vi "Init.vi"(8 "error in":errorcluster, 10 "File Path":path, 11 "XLS in":refnum<class "XLS.lvclass">) -> (0 "error out":errorcluster, 3 "XLS out":refnum<class "XLS.lvclass">)   [LabVIEW 2017, in "Report_lib.lvlib" / "XLS.lvclass"]
doc: "This method serves for Creating XLS file\nand Generate its filename"
uses:
  XLS.lvclass
  I:/TEMP/Source/Classes/Log/Log.lvclass
  Log/Log.lvclass/Log.ctl
  XLS.lvclass/XLS.ctl
  Log/Log.lvclass
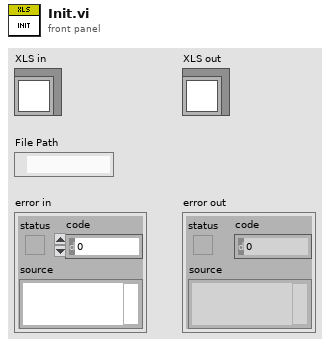
[diagram p1: front panel]
types:
  T1 = typedef "Log Data.ctl" = cluster{"File Path":path, "File Name":string, "File Ext":string}
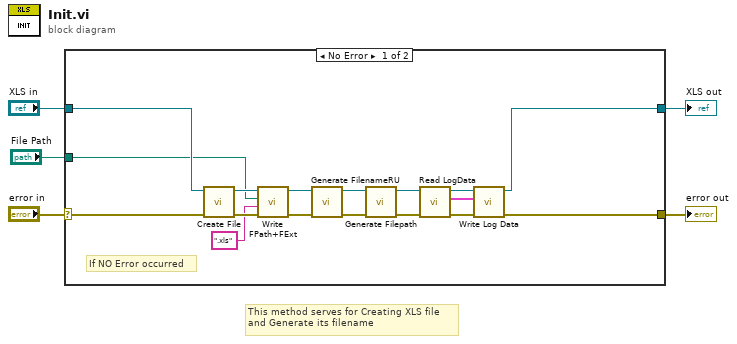
[diagram p0: block diagram]
diagram:
  # "This method serves for Creating XLS file\nand Generate its filename"
  n1 = case shown="No Error" "error in" {
    selector: "error in" -> [w20 w24]
    tunnel: [w8 w24] -> w4
    tunnel: [w9 w23] -> w2
    tunnel: "XLS in" -> [w22 w23]
    tunnel: "File Path" -> [w6 _]
    frame No Error {
      # "If NO Error occurred"
      n2 = call-dynamic "Create File.vi"("error in"=w20, "XLS in"=w22) -> ("error out"=w19:errorcluster, "XLS out"=w21:refnum<class "XLS.lvclass">)  [unwired: 8 in]
      n3 = call "Write FPath+FExt.vi"("error in (no error)"=w19, "File Ext"=".xls", "File Path"=w6, "Log in"=w21) -> ("error out"=w18:errorcluster, "Log out"=w17:refnum<class "XLS.lvclass">)  [unwired: 6 in]
      n4 = call "Generate FilenameRU.vi"("error in"=w18, "Log in"=w17) -> ("error out"=w16:errorcluster, "Log out"=w15:refnum<class "XLS.lvclass">)  [unwired: 8 in]
      n5 = call "Generate Filepath.vi"("error in"=w16, "Log in"=w15) -> ("error out"=w13:errorcluster, "Log out"=w14:refnum<class "XLS.lvclass">)  [unwired: 8 in]
      n6 = call "Read LogData.vi"("error in (no error)"=w13, "Log in"=w14) -> ("error out"=w12:errorcluster, "Log Data"=w10:T1, "Log out"=w11:refnum<class "XLS.lvclass">)  [unwired: 7 in]
      n7 = call "Write Log Data.vi"("error in"=w12, "Log Data"=w10, "XLS in"=w11) -> ("error out"=w8:errorcluster, "XLS out"=w9:refnum<class "XLS.lvclass">)  [unwired: 7 in]
    }
    frame Error {
    }
  }
  "error out" <- w4
  "XLS out" <- w2
